vi "ProgressBar close.vi"(8 "error in (no error)":errorcluster, 11 "ProgressBar in":refnum<class "ProgressBar.lvclass">) -> (0 "error out":errorcluster, 3 "ProgressBar out":refnum<class "ProgressBar.lvclass">)   [LabVIEW 2018, in "ProgressBar.lvclass"]
uses:
  ProgressBar.lvclass
  ProgressBar.lvclass/ProgressBar.ctl
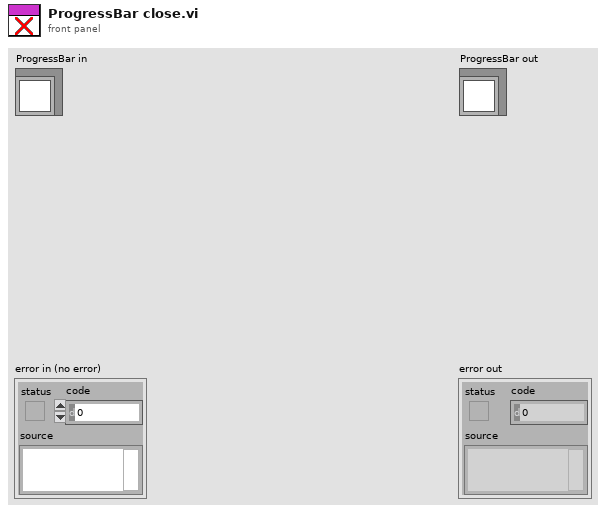
[diagram p1: front panel]
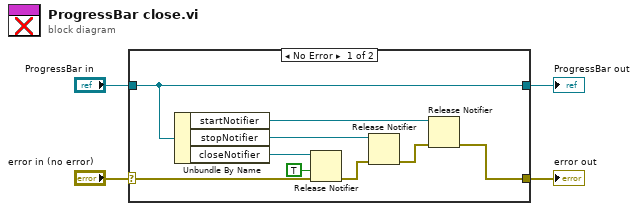
[diagram p0: block diagram]
diagram:
  n1 = case shown="No Error" "error in (no error)" {
    selector: "error in (no error)" -> [w6 w15]
    tunnel: [w5 w15] -> w3
    tunnel: [w13 w14] -> w1
    tunnel: "ProgressBar in" -> [w13 w14]
    frame No Error {
      n2 = Unbundle By Name(w13) -> ("startNotifier"=w10:refnum<notifier>, "stopNotifier"=w11:refnum<notifier>, "closeNotifier"=w12:refnum<notifier>)
      n3 = Release Notifier(notifier=w12, force destroy? (F)=TRUE, error in (no error)=w6) -> (error out=w8:errorcluster)  [unwired: 2 out]
      n4 = Release Notifier(notifier=w11, error in (no error)=w8) -> (error out=w7:errorcluster)  [unwired: 1 in, 2 out]
      n5 = Release Notifier(notifier=w10, error in (no error)=w7) -> (error out=w5:errorcluster)  [unwired: 1 in, 2 out]
    }
    frame Error {
    }
  }
  "error out" <- w3
  "ProgressBar out" <- w1
